vi "VisionGlobals.vi"() -> ()   [LabVIEW 2015]
panel:
  out "AutoTargetEnabled?":bool
  out "LEDOutput":u16
  out "FlipImage":bool
  out "LastValueCOM":dbl
  out "LastValueArea":dbl
  out "OnTarget?":bool
  out "DriveEnabled?":bool
  out "CenterOfMassX":dbl
  out "NumberOfParticles":dbl
  out "ParticleWidth":dbl
  out "FirstPixelX":dbl
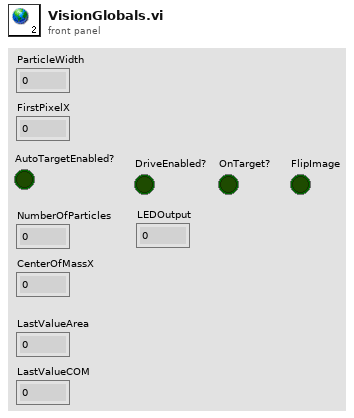
[diagram p1: front panel]
diagram:
